vi "DataExcelFileRichInfo.vi"(9 "Language":u32, 11 "file path (dialog if empty)":path caption="文件路径 （空时为对话框）") -> (0 "路径输出":path, 1 "FileInfo":string, 2 "文件类型":string)   [LabVIEW 2015]
uses:
  <vilib>/addons/_office/excel.llb/Excel Get Data ([str]).vi
  <vilib>/Utility/NIReport.llb/NI_report.lvclass
  <vilib>/addons/_office/NI_ReportGenerationToolkit.lvlib
  <vilib>/Utility/NIReport.llb/Excel/NI_Excel.lvclass
panel:
  out "判断":string
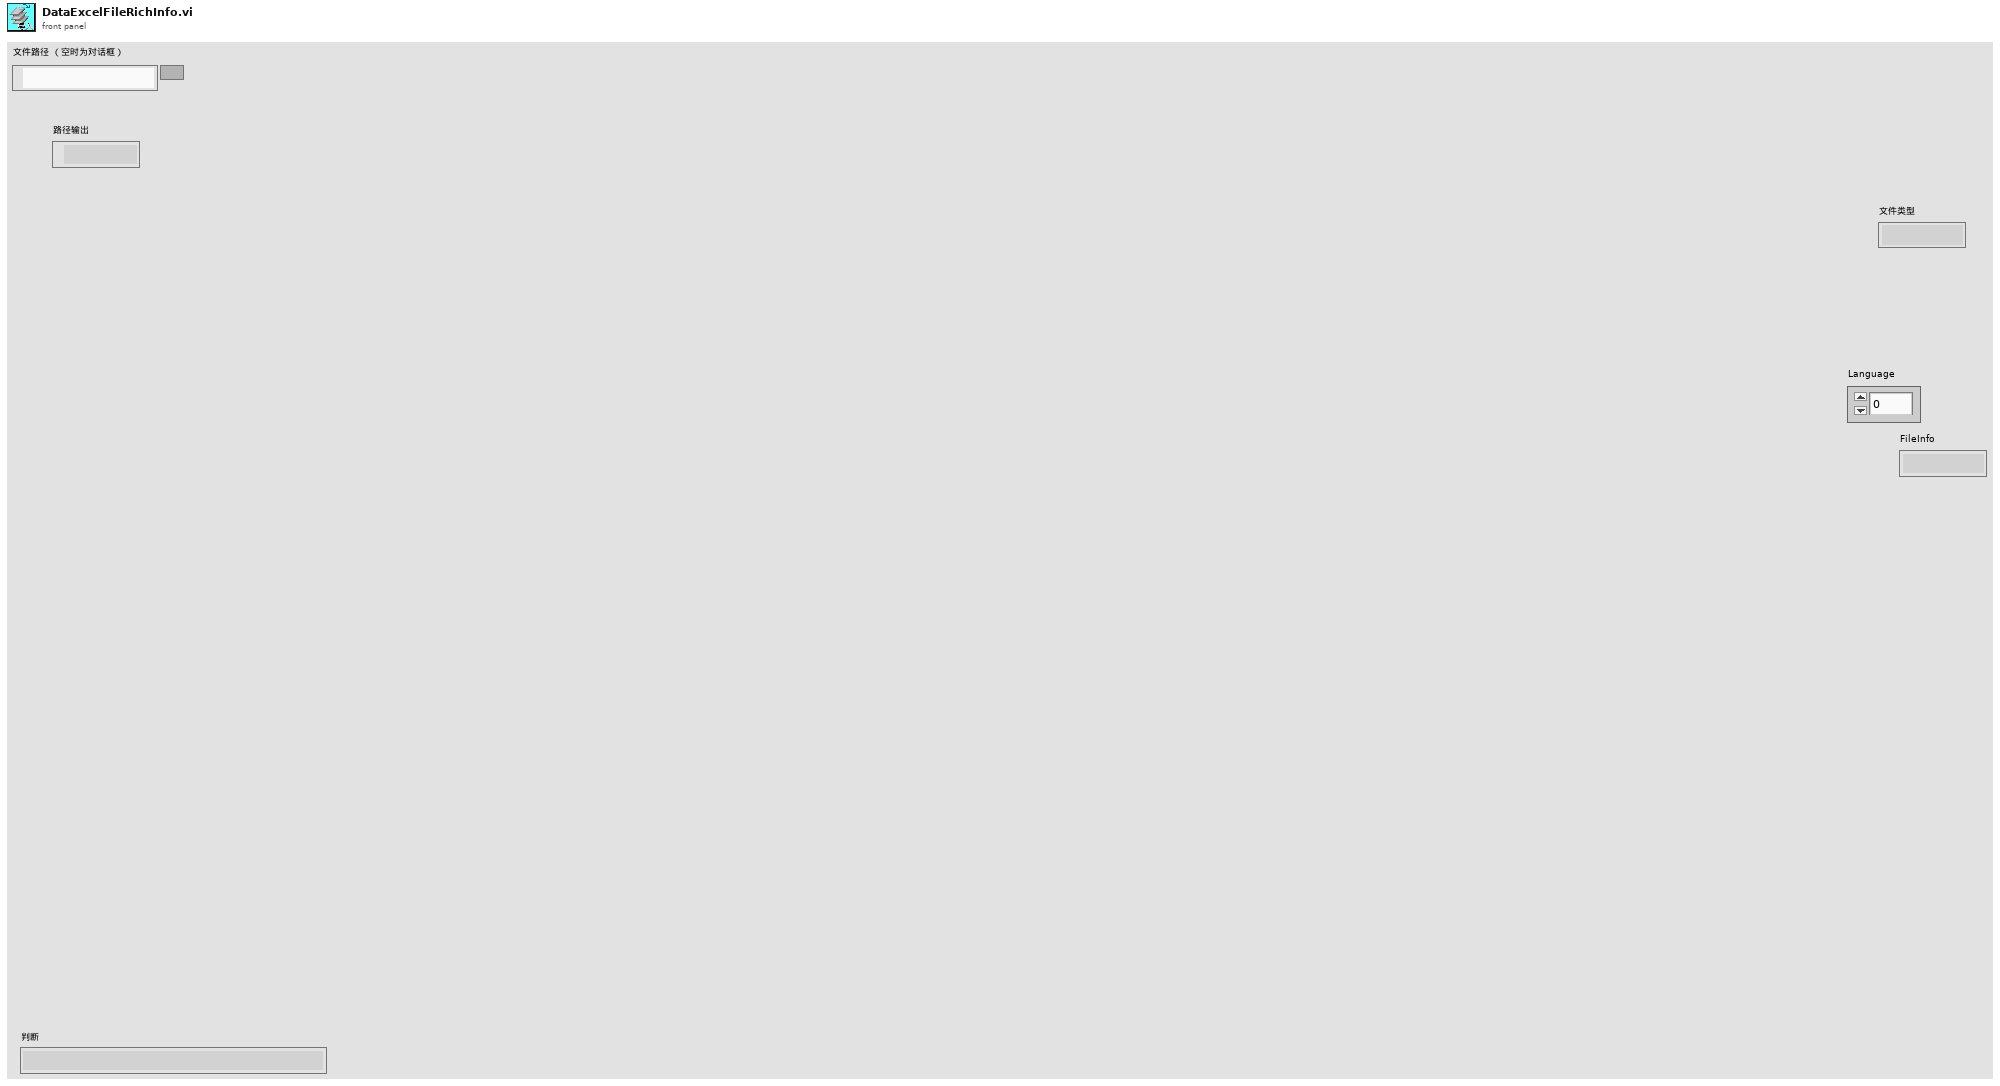
[diagram p1: front panel]
types:
  T1 = enum16{"maximized", "minimized", "normal", "no change"}
  T2 = enum16{"Standard Report", "HTML", "Word", "Excel"}
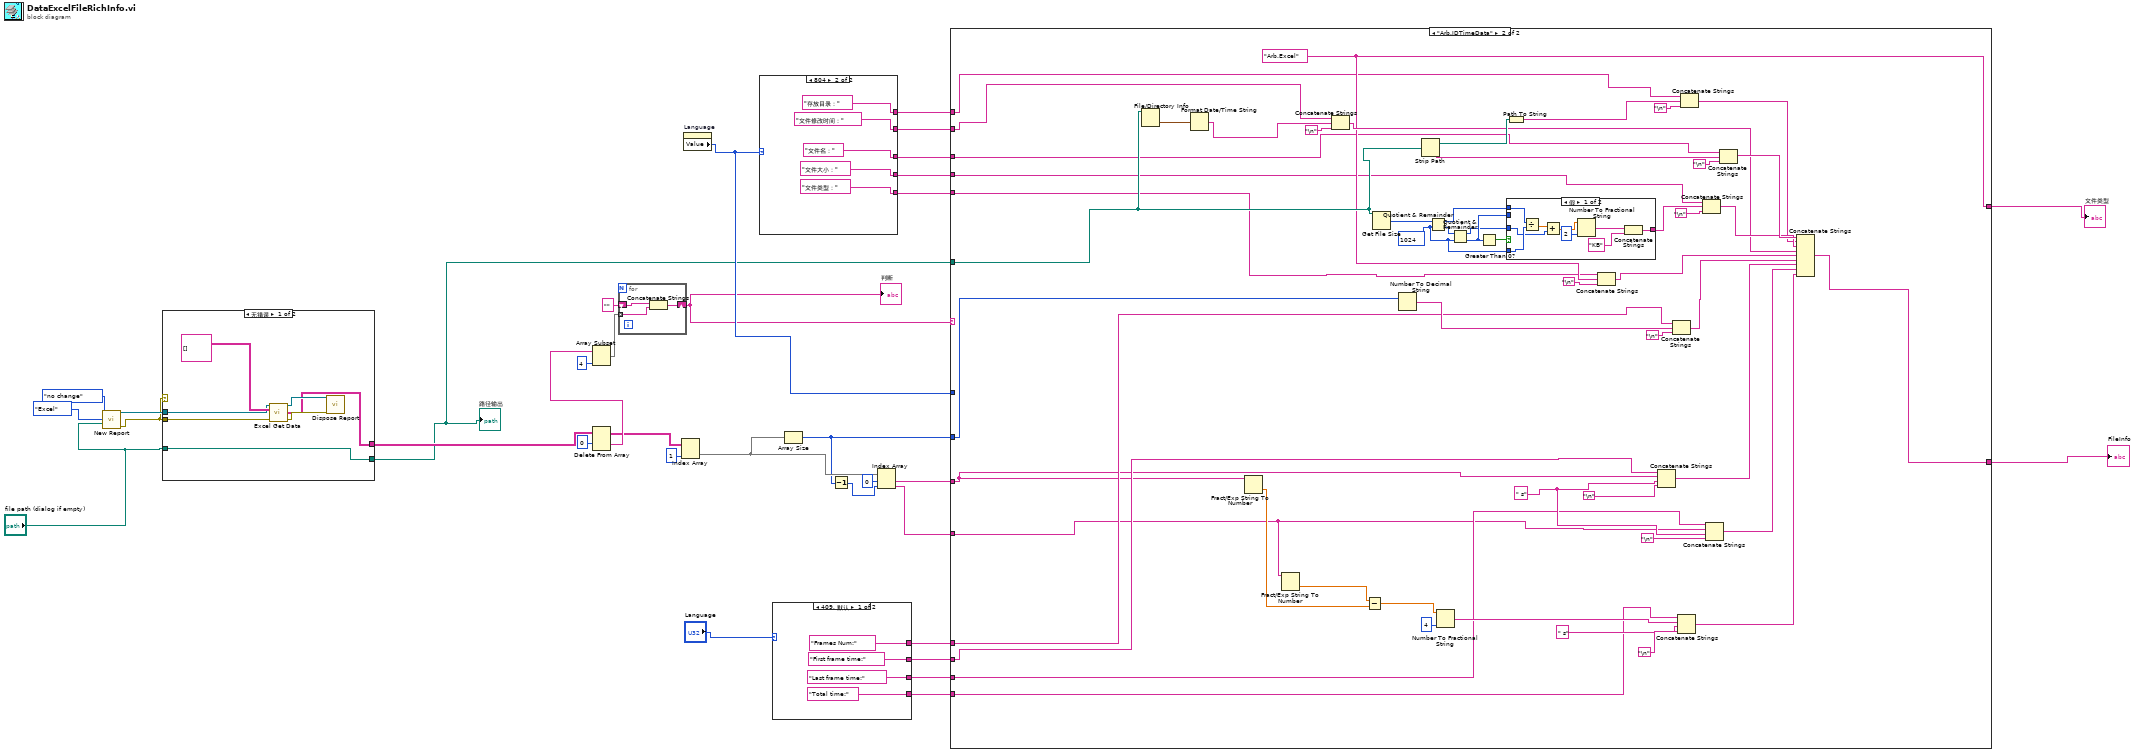
[diagram p0: block diagram]
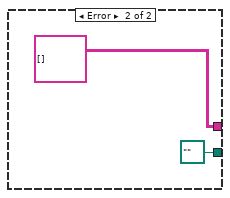
[diagram p2: hidden frame]
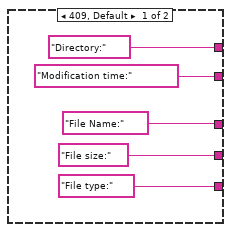
[diagram p3: hidden frame]
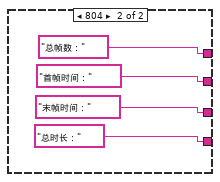
[diagram p4: hidden frame]
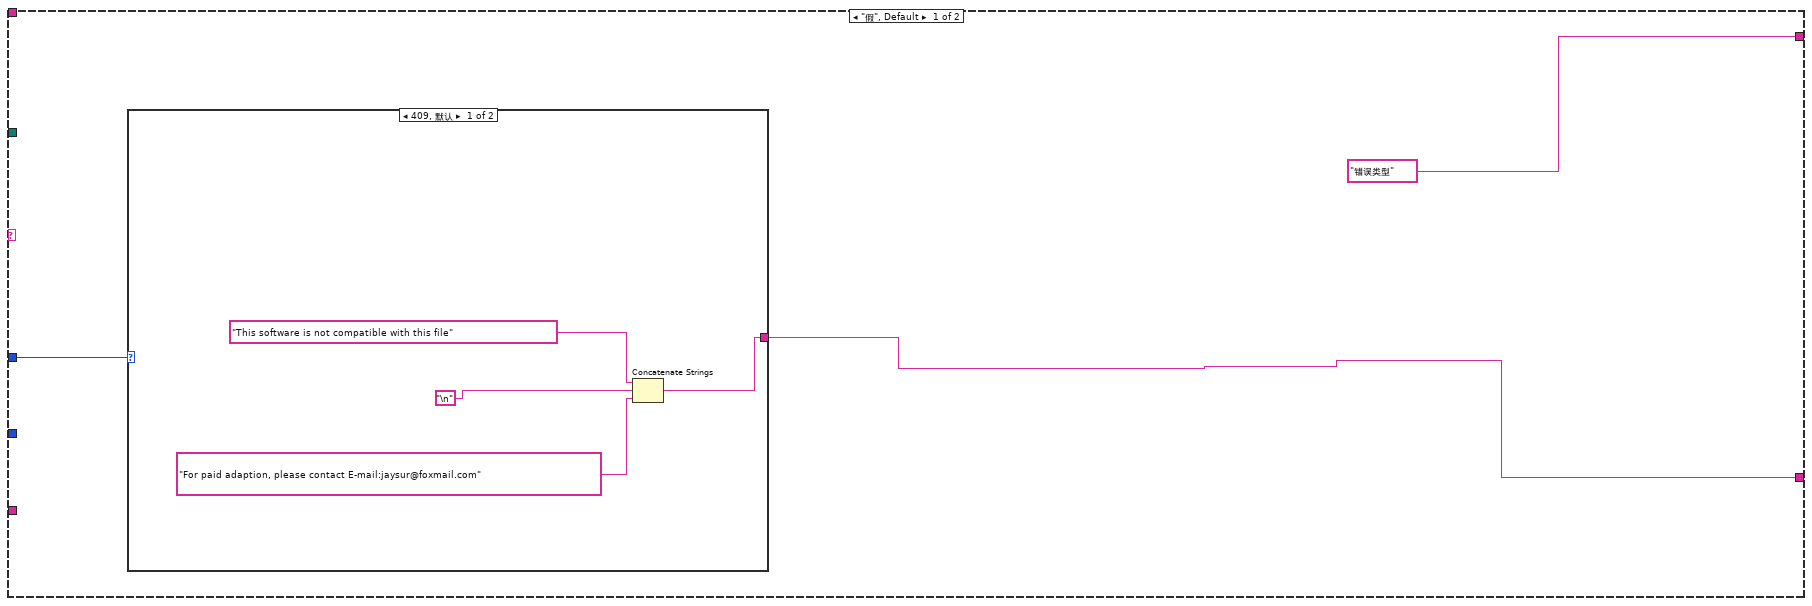
[diagram p5: hidden frame]
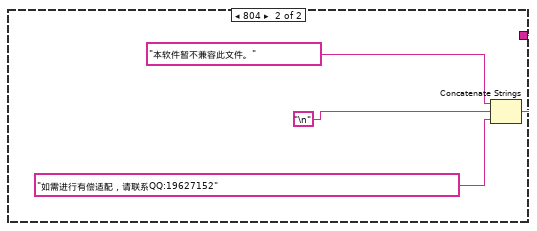
[diagram p6: hidden frame]
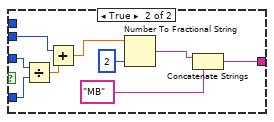
[diagram p7: hidden frame]
diagram:
  n1 = call <vilib>:"New Report.vi"("window state (normal)"=T1."no change", "report type"=T2."Excel", "template (empty)"="file path (dialog if empty)") -> ("report out"=w21:refnum<class "NI_report.lvclass">, "error out"=w18:errorcluster)  [unwired: 11 in]
  n2 = case shown="无错误" w18 {
    tunnel: w21 -> [w40 _]
    tunnel: w18 -> [w39 _]
    tunnel: [w36 string[][] []] -> w11
    tunnel: "file path (dialog if empty)" -> [w35 _]
    tunnel: [w35 path "" ("file path (dialog if empty)")] -> w10
    frame No Error {
      n3 = call-poly <vilib>:"Excel Get Data.vi"("report in"=w40, "data type"=string[][] [], "error in (no error)"=w39) -> ("report out"=w37:refnum<class "NI_report.lvclass">, "data"=w36:string[][], "error out"=w38:errorcluster)  [unwired: 10 in]
      n4 = call-dynamic "Dispose Report.vi"("report in"=w37, "error in (no error)"=w38) -> ()  [unwired: 13 in, 1 out]
    }
    frame Error {
    }
  }
  "路径输出" <- w10
  n5 = Delete From Array(array=w11, index (row)=0 ("索引 (行)")) -> (deleted portion=w12:string[], array with subset deleted=w8:string[][])  [unwired: 2 in]
  n6 = Array Subset(array=w12, length=4 ("长度")) -> (w13:string[])  [unwired: 1 in]
  n7 = for {
    tunnel: w13 -> [w45] mode=indexing
    shift-right: [w46] -> w9
    shift-left: "" -> [w44]
    n8 = Concatenate Strings(w44, w45) -> (w46:string)
  }
  "判断" <- w9
  n9 = Index Array(array=w8, index (col)=1 ("禁用的索引 (列)")) -> (element=w6:string[])  [unwired: 1 in]
  n10 = property on="Language" class="DigNum (严格)"() -> ("Value"=w31:u32)  [unwired: 2 in, 2 out]
  n11 = case shown="804" w31 {
    tunnel: ["Modification time:" "文件修改时间："] -> w29
    tunnel: ["Directory:" "存放目录："] -> w30
    tunnel: ["File Name:" "文件名："] -> w28
    tunnel: ["File size:" "文件大小："] -> w27
    tunnel: ["File type:" "文件类型："] -> w26
    frame 409, Default {
    }
    frame 804 {
    }
  }
  n12 = case shown="409, 默认" "Language" {
    tunnel: ["Total time:" "总时长："] -> w25
    tunnel: ["Last frame time:" "末帧时间："] -> w24
    tunnel: ["First frame time:" "首帧时间："] -> w23
    tunnel: ["Frames Num:" "总帧数："] -> w22
    frame 409, Default {
    }
    frame 804 {
    }
  }
  n13 = Array Size(array=w6) -> (size(s)=w4:i32)
  n14 = Decrement(x=w4) -> (x-1=w3:i32)
  n15 = Index Array(array=w6, index #1=0 ("索引"), index #2=w3) -> (element #1=w1:string, element #2=w2:string)
  n16 = case shown="\"Arb.IDTimeData\"" w9 {
    tunnel: ["错误类型" w88] -> w34
    tunnel: [w66 w111] -> w33
    tunnel: w10 -> [_ w103]
    tunnel: w31 -> [w65 _]
    tunnel: w30 -> [_ w84]
    tunnel: w29 -> [_ w83]
    tunnel: w28 -> [_ w85]
    tunnel: w27 -> [_ w86]
    tunnel: w26 -> [_ w87]
    tunnel: w25 -> [_ w79]
    tunnel: w24 -> [_ w80]
    tunnel: w23 -> [_ w82]
    tunnel: w22 -> [_ w81]
    tunnel: w4 -> [_ w78]
    tunnel: w2 -> [_ w77]
    tunnel: w1 -> [_ w76]
    frame "假", Default {
      n17 = case shown="409, 默认" w65 {
        tunnel: [w68 w72] -> w66
        frame 409, Default {
          n18 = Concatenate Strings("This software is not compatible with this file", "\n", "For paid adaption, please contact E-mail:jaysur@foxmail.com") -> (w68:string)
        }
        frame 804 {
          n19 = Concatenate Strings("本软件暂不兼容此文件。", "\n", "如需进行有偿适配，请联系QQ:19627152") -> (w72:string)
        }
      }
    }
    frame "Arb.IDTimeData" {
      w98 = " s"
      w116 = i64 1024 ("y")
      w88 = "Arb.Excel"
      n20 = File/Directory Info(path=w103) -> (last mod=w106:timestamp)  [unwired: 1 in, 6 out]
      n21 = Format Date/Time String(seconds (now)=w106) -> (date/time string=w104:string)  [unwired: 2 in]
      n22 = Fract/Exp String To Number(string=w76) -> (number=w96:dbl)  [unwired: 3 in, 1 out]
      n23 = Fract/Exp String To Number(string=w77) -> (number=w97:dbl)  [unwired: 3 in, 1 out]
      n24 = Concatenate Strings(w83, w104, "\n") -> (w102:string)
      n25 = Subtract(x=w97, y=w96) -> (x-y=w95:dbl)
      n26 = Get File Size(file=w103) -> (size (in bytes)=w119:i64)  [unwired: 1 in, 2 out]
      n27 = Number To Decimal String(number=w78) -> (decimal integer string=w122:string)  [unwired: 1 in]
      n28 = Strip Path(path=w103) -> (stripped path=w108:path, name=w129:string)
      n29 = Quotient & Remainder(x=w119, y=w116) -> (x-y*floor(x/y)=w112:i64, floor(x/y)=w118:i64)
      n30 = Number To Fractional String(number=w95, precision (6)=i16 4 ("精度(6)")) -> (F-format string=w93:string)  [unwired: 2 in]
      n31 = Quotient & Remainder(x=w118, y=w116) -> (x-y*floor(x/y)=w114:i64, floor(x/y)=w115:i64)
      n32 = Greater Than 0?(x=w115) -> (x > 0?=w117:bool)
      n33 = case shown="假" w117 {
        tunnel: w116 -> [w135 w145]
        tunnel: w115 -> [_ w143]
        tunnel: w114 -> [w133 w146]
        tunnel: [w138 w141] -> w113
        tunnel: w112 -> [w136 _]
        frame False {
          n34 = Divide(x=w136, y=w135) -> (x/y=w134:dbl)
          n35 = Add(x=w134, y=w133) -> (x+y=w132:dbl)
          n36 = Number To Fractional String(number=w132, precision (6)=i16 2 ("精度(6)")) -> (F-format string=w130:string)  [unwired: 2 in]
          n37 = Concatenate Strings(w130, "KB" ("字符串")) -> (w138:string)
        }
        frame True {
          n38 = Divide(x=w146, y=w145) -> (x/y=w144:dbl)
          n39 = Add(x=w143, y=w144) -> (x+y=w142:dbl)
          n40 = Number To Fractional String(number=w142, precision (6)=i16 2 ("精度(6)")) -> (F-format string=w140:string)  [unwired: 2 in]
          n41 = Concatenate Strings(w140, "MB") -> (w141:string)
        }
      }
      n42 = Path To String(path=w108) -> (string=w109:string)
      n43 = Concatenate Strings(w87, w88, "\n") -> (w126:string)
      n44 = Concatenate Strings(w82, w76, w98, "\n") -> (w91:string)
      n45 = Concatenate Strings(w81, w122, "\n") -> (w123:string)
      n46 = Concatenate Strings(w79, w93, " s", "\n") -> (w89:string)
      n47 = Concatenate Strings(w84, w109, "\n") -> (w107:string)
      n48 = Concatenate Strings(w86, w113, "\n") -> (w120:string)
      n49 = Concatenate Strings(w80, w77, w98, "\n") -> (w90:string)
      n50 = Concatenate Strings(w85, w129, "\n") -> (w128:string)
      n51 = Concatenate Strings(w128, w107, w120, w102, w126, w123, w91, w90, w89) -> (w111:string)
    }
  }
  "FileInfo" <- w33
  "文件类型" <- w34
